vi "Tosca-Create DI File Header.vi"(0 "Digital Inputs":T5[](array[typedef]), 7 "Input Events":T1[](array[typedef])) -> (4 "DI Write Order":i32[](array[numeric]), 6 "Num Columns":i32, 8 "header":string)   [LabVIEW 2020]
uses:
  Tosca-Digital Input.ctl
  Tosca-Input Event.ctl
  Tosca-Input Criterion.ctl
  epl-vi-lib/Utility VIs/Type Defs/Logic State.ctl
  Typedefs/Tosca-Accumulator.ctl
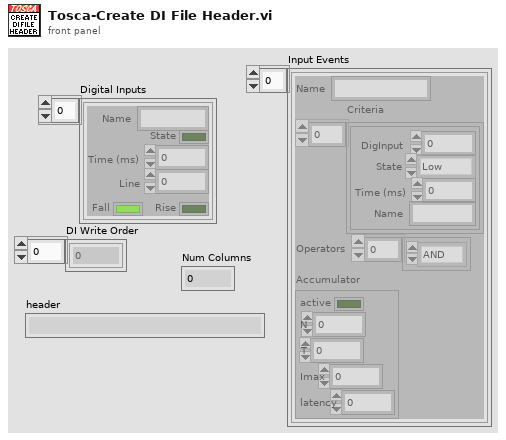
[diagram p1: front panel]
types:
  T1 = typedef "Tosca-Input Event.ctl" = cluster{"Name":string, "Criteria":T2[], "Operators":enum16{"AND", "OR"}[], "Accumulator":T4}
  T2 = typedef "Tosca-Input Criterion.ctl" = cluster{"DigInput":i32, "State":T3, "Time (ms)":i32, "Name":string}
  T3 = typedef "Logic State.ctl" = enum16{"Low", "High", "Rising", "Falling"}
  T4 = typedef "Tosca-Accumulator.ctl" = cluster{"active":bool, "N":i32, "T":dbl, "Imax":dbl, "latency":dbl}
  T5 = typedef "Tosca-Digital Input.ctl" = cluster{"Name":string, "State":bool, "Time (ms)":dbl, "Line":i32, "Rise":bool, "Fall":bool}
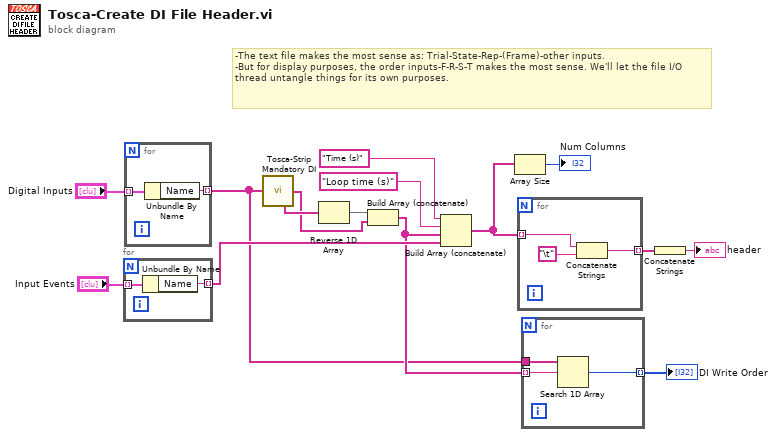
[diagram p0: block diagram]
diagram:
  # "-The text file makes the most sense as: Trial-State-Rep-(Frame)-other inputs.\n-But for display purposes, the order inputs-F-R-S-T makes the most sense. We'll let the file I/O thread untangle things for its own purposes."
  n1 = for {
    tunnel: "Input Events" -> [w17] mode=indexing
    tunnel: [w16] -> w15 mode=indexing
    n2 = Unbundle By Name(w17) -> ("Name"=w16:string)
  }
  n3 = for {
    tunnel: "Digital Inputs" -> [w19] mode=indexing
    tunnel: [w18] -> w3 mode=indexing
    n4 = Unbundle By Name(w19) -> ("Name"=w18:string)
  }
  n5 = call "Tosca-Strip Mandatory DI.vi"("Digital Signals"=w3) -> ("Filtered DI"=w5:string[], "Required"=w10:string[])  [unwired: 12 in, 1 out]
  n6 = Reverse 1D Array(array=w10) -> (reversed array=w6:string[])
  n7 = Build Array (concatenate)(w6, w5) -> (w4:string[])
  n8 = Build Array (concatenate)("Time (s)", "Loop time (s)", w4, w15) -> (w8:string[])
  n9 = Array Size(array=w8) -> (size(s)=→"Num Columns":i32)
  n10 = for {
    tunnel: w8 -> [w20] mode=indexing
    tunnel: [w22] -> w12 mode=indexing
    n11 = Concatenate Strings(w20, "\t") -> (w22:string)
  }
  n12 = for {
    tunnel: w4 -> [w24] mode=indexing
    tunnel: w3 -> [w25]
    tunnel: [w23] -> w2 mode=indexing
    n13 = Search 1D Array(1D array=w25, element=w24) -> (index of element=w23:i32)  [unwired: 1 in]
  }
  "DI Write Order" <- w2
  n14 = Concatenate Strings(w12) -> (→"header":string)
